vi "commandes manuelles 2 axes.vi"() -> ()   [LabVIEW 2016]
uses:
  Variable globale.vi
panel:
  in  "RETOUR":bool
  in  "Vitesse Manuelle en mm/s":dbl(slide) scale=0.0..1000.0
  in  "x+y-":bool
  in  "x-y-":bool
  in  "x-y+":bool
  in  "x+y+":bool
  in  "y-":bool
  in  "y+":bool
  in  "x-":bool
  in  "x+":bool
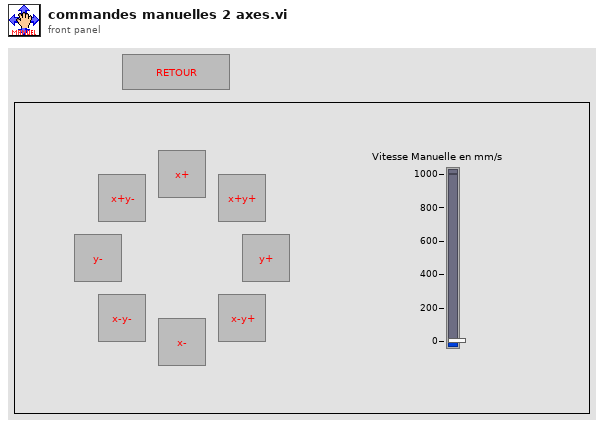
[diagram p1: front panel]
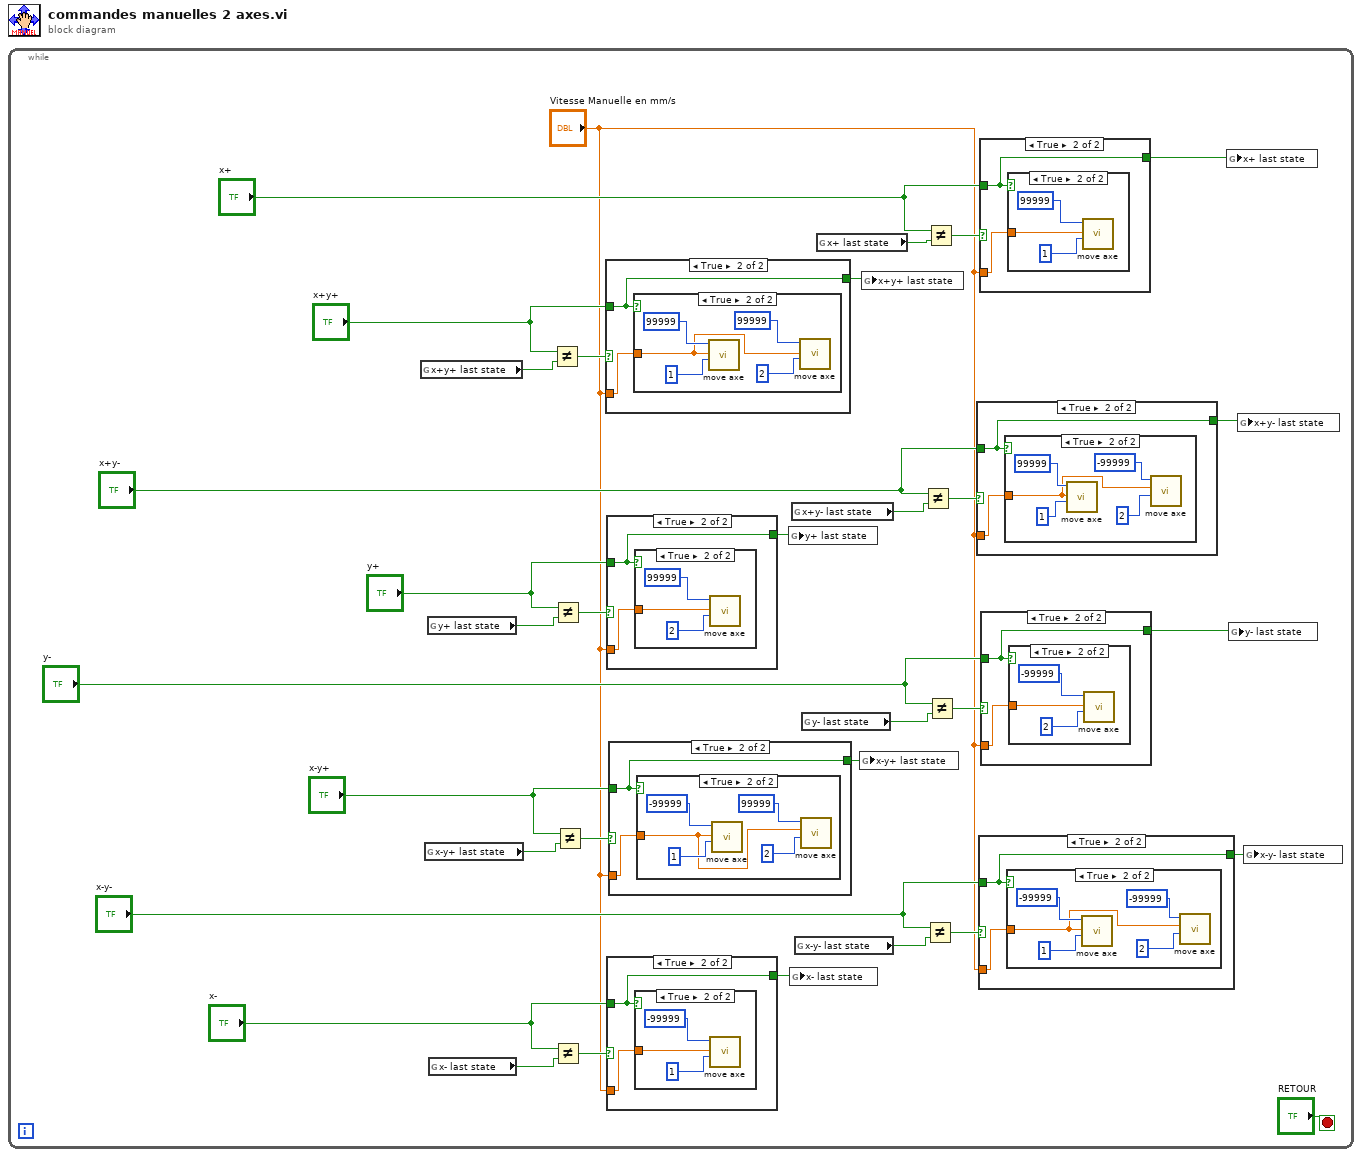
[diagram p0: block diagram]
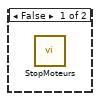
[diagram p3: hidden frame]
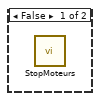
[diagram p5: hidden frame]
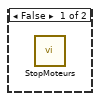
[diagram p7: hidden frame]
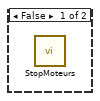
[diagram p9: hidden frame]
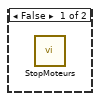
[diagram p11: hidden frame]
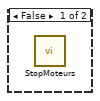
[diagram p13: hidden frame]
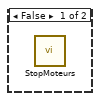
[diagram p15: hidden frame]
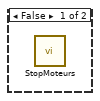
[diagram p17: hidden frame]
diagram:
  n1 = while {
    stop <- "RETOUR" stop-if-true
    n2 = global read "Variable globale.vi" "x+y+ last state"() -> (w29:bool)
    n3 = global read "Variable globale.vi" "x-y+ last state"() -> (w13:bool)
    n4 = global read "Variable globale.vi" "y+ last state"() -> (w21:bool)
    n5 = global read "Variable globale.vi" "x- last state"() -> (w25:bool)
    n6 = Not Equal?(x="x+y+", y=w29) -> (x != y?=w30:bool)
    n7 = Not Equal?(x="y+", y=w21) -> (x != y?=w22:bool)
    n8 = Not Equal?(x="x-", y=w25) -> (x != y?=w26:bool)
    n9 = Not Equal?(x="x-y+", y=w13) -> (x != y?=w14:bool)
    n10 = case shown="True" w30 {
      tunnel: "Vitesse Manuelle en mm/s" -> [_ w79]
      tunnel: "x+y+" -> [w77 w78]
      tunnel: [w77 w78] -> w28
      frame False {
      }
      frame True {
        n11 = case shown="True" w78 {
          tunnel: w79 -> [_ w81]
          frame False {
            n12 = call "StopMoteurs.vi"() -> ()  [unwired: 12 in]
          }
          frame True {
            n13 = call "move axe.vi"("Axe"=1, "Vitesse"=w81, "Angle"=99999) -> ()  [unwired: 9 in]
            n14 = call "move axe.vi"("Axe"=2, "Vitesse"=w81, "Angle"=99999) -> ()  [unwired: 9 in]
          }
        }
      }
    }
    n15 = case shown="True" w22 {
      tunnel: "Vitesse Manuelle en mm/s" -> [_ w67]
      tunnel: "y+" -> [w65 w66]
      tunnel: [w65 w66] -> w20
      frame False {
      }
      frame True {
        n16 = case shown="True" w66 {
          tunnel: w67 -> [_ w69]
          frame False {
            n17 = call "StopMoteurs.vi"() -> ()  [unwired: 12 in]
          }
          frame True {
            n18 = call "move axe.vi"("Axe"=2, "Vitesse"=w69, "Angle"=99999) -> ()  [unwired: 9 in]
          }
        }
      }
    }
    n19 = case shown="True" w26 {
      tunnel: "Vitesse Manuelle en mm/s" -> [_ w73]
      tunnel: "x-" -> [w71 w72]
      tunnel: [w71 w72] -> w24
      frame False {
      }
      frame True {
        n20 = case shown="True" w72 {
          tunnel: w73 -> [_ w75]
          frame False {
            n21 = call "StopMoteurs.vi"() -> ()  [unwired: 12 in]
          }
          frame True {
            n22 = call "move axe.vi"("Axe"=1, "Vitesse"=w75, "Angle"=-99999) -> ()  [unwired: 9 in]
          }
        }
      }
    }
    n23 = case shown="True" w14 {
      tunnel: "Vitesse Manuelle en mm/s" -> [_ w51]
      tunnel: "x-y+" -> [w49 w50]
      tunnel: [w49 w50] -> w12
      frame False {
      }
      frame True {
        n24 = case shown="True" w50 {
          tunnel: w51 -> [_ w52]
          frame False {
            n25 = call "StopMoteurs.vi"() -> ()  [unwired: 12 in]
          }
          frame True {
            n26 = call "move axe.vi"("Axe"=1, "Vitesse"=w52, "Angle"=-99999) -> ()  [unwired: 9 in]
            n27 = call "move axe.vi"("Axe"=2, "Vitesse"=w52, "Angle"=99999) -> ()  [unwired: 9 in]
          }
        }
      }
    }
    n28 = global write "Variable globale.vi" "y+ last state"(w20) -> ()
    n29 = global write "Variable globale.vi" "x- last state"(w24) -> ()
    n30 = global read "Variable globale.vi" "x+y- last state"() -> (w17:bool)
    n31 = global read "Variable globale.vi" "x-y- last state"() -> (w5:bool)
    n32 = global read "Variable globale.vi" "y- last state"() -> (w9:bool)
    n33 = global read "Variable globale.vi" "x+ last state"() -> (w33:bool)
    n34 = global write "Variable globale.vi" "x-y+ last state"(w12) -> ()
    n35 = global write "Variable globale.vi" "x+y+ last state"(w28) -> ()
    n36 = Not Equal?(x="x+y-", y=w17) -> (x != y?=w18:bool)
    n37 = Not Equal?(x="x-y-", y=w5) -> (x != y?=w6:bool)
    n38 = Not Equal?(x="x+", y=w33) -> (x != y?=w34:bool)
    n39 = Not Equal?(x="y-", y=w9) -> (x != y?=w10:bool)
    n40 = case shown="True" w18 {
      tunnel: "Vitesse Manuelle en mm/s" -> [_ w59]
      tunnel: "x+y-" -> [w57 w58]
      tunnel: [w57 w58] -> w16
      frame False {
      }
      frame True {
        n41 = case shown="True" w58 {
          tunnel: w59 -> [_ w60]
          frame False {
            n42 = call "StopMoteurs.vi"() -> ()  [unwired: 12 in]
          }
          frame True {
            n43 = call "move axe.vi"("Axe"=1, "Vitesse"=w60, "Angle"=99999) -> ()  [unwired: 9 in]
            n44 = call "move axe.vi"("Axe"=2, "Vitesse"=w60, "Angle"=-99999) -> ()  [unwired: 9 in]
          }
        }
      }
    }
    n45 = case shown="True" w6 {
      tunnel: "Vitesse Manuelle en mm/s" -> [_ w37]
      tunnel: "x-y-" -> [w35 w36]
      tunnel: [w35 w36] -> w4
      frame False {
      }
      frame True {
        n46 = case shown="True" w36 {
          tunnel: w37 -> [_ w38]
          frame False {
            n47 = call "StopMoteurs.vi"() -> ()  [unwired: 12 in]
          }
          frame True {
            n48 = call "move axe.vi"("Axe"=1, "Vitesse"=w38, "Angle"=-99999) -> ()  [unwired: 9 in]
            n49 = call "move axe.vi"("Axe"=2, "Vitesse"=w38, "Angle"=-99999) -> ()  [unwired: 9 in]
          }
        }
      }
    }
    n50 = case shown="True" w34 {
      tunnel: "Vitesse Manuelle en mm/s" -> [_ w87]
      tunnel: "x+" -> [w85 w86]
      tunnel: [w85 w86] -> w32
      frame False {
      }
      frame True {
        n51 = case shown="True" w86 {
          tunnel: w87 -> [_ w89]
          frame False {
            n52 = call "StopMoteurs.vi"() -> ()  [unwired: 12 in]
          }
          frame True {
            n53 = call "move axe.vi"("Axe"=1, "Vitesse"=w89, "Angle"=99999) -> ()  [unwired: 9 in]
          }
        }
      }
    }
    n54 = case shown="True" w10 {
      tunnel: "Vitesse Manuelle en mm/s" -> [_ w45]
      tunnel: "y-" -> [w43 w44]
      tunnel: [w43 w44] -> w8
      frame False {
      }
      frame True {
        n55 = case shown="True" w44 {
          tunnel: w45 -> [_ w47]
          frame False {
            n56 = call "StopMoteurs.vi"() -> ()  [unwired: 12 in]
          }
          frame True {
            n57 = call "move axe.vi"("Axe"=2, "Vitesse"=w47, "Angle"=-99999) -> ()  [unwired: 9 in]
          }
        }
      }
    }
    n58 = global write "Variable globale.vi" "x+ last state"(w32) -> ()
    n59 = global write "Variable globale.vi" "y- last state"(w8) -> ()
    n60 = global write "Variable globale.vi" "x+y- last state"(w16) -> ()
    n61 = global write "Variable globale.vi" "x-y- last state"(w4) -> ()
  }
